vi "Server_Globals.vi"() -> ()   [LabVIEW 2011]
doc: "The Server_Globals vi contain global variables used within the server software."
panel:
  out "External Settings":T1
  in  "Session Settings":T2={"I/O Settings"=[0, 0, 0, 0, 0, 0, 0, 0, 0, 0, 0, 0, 0, 0, 0, 0, 0], "Instrument Handle"={"5402"="", " 5112"="", "4072"="", "USB"="", "4110"=""}, "Logfile"=refnum, "Log Level"=0, "Clear"=[], "OS Set"={"instrument handle out"="", "remaining string"="", "Settings"={"Horizontal Conf."={"Min. Sample rate"=0.0, "Reference position"=0.0, "Record Length"=0}, "Channel A"={"Enable"=FALSE, "Vertical coupling"=0.0, "Vertical range"=0.0, "Vertical offset"=0.0, "Probe attenuation"=1.0}, "Channel B"={"Enable"=FALSE, "Vertical coupling"=0.0, "Vertical range"=0.0, "Vertical offset"=0.0, "Probe attenuation"=1.0}, "Trigger"={"Source"=enum."channel 1", "Slope"=enum."Positive", "Coupling"=enum."AC", "Level"=0.0, "Holdoff"=0.0, "Delay"=0.0, " Timeout"=0.0, " Mode"=enum."Normal"}, "Measurements"={"Measurement 1, Channel"=enum."Channel 1", "Measurement 1, Selection"=0, "Measurement 2, Channel"=enum."Channel 1", "Measurement 2,  Selection"=0, "Measurement 3, Channel"=enum."Channel 1", "Measurement 3, Selection 3"=0}}}, "DC Power Supply"={"0"="", "1"="", "2"="", "3"="", "4"=""}, "USB Interface"={"0"="", "1"="", "2"="", "3"="", "4"=""}, "Function Generator"={"0"="", "1"="", "2"="", "3"="", "4"=""}, "Digital Multimeter"={"0"="", "1"="", "2"="", "3"="", "4"=""}, "Digital Osciliscope"={"0"="", "1"="", "2"="", "3"="", "4"=""}, "To M Server"="", "Adres"=[], "Matrix version"="", "MD5"="", "Digital Multimeter Card 2"={"0"="", "1"="", "2"="", "3"="", "4"=""}} {"I/O Settings" format="%032b"}
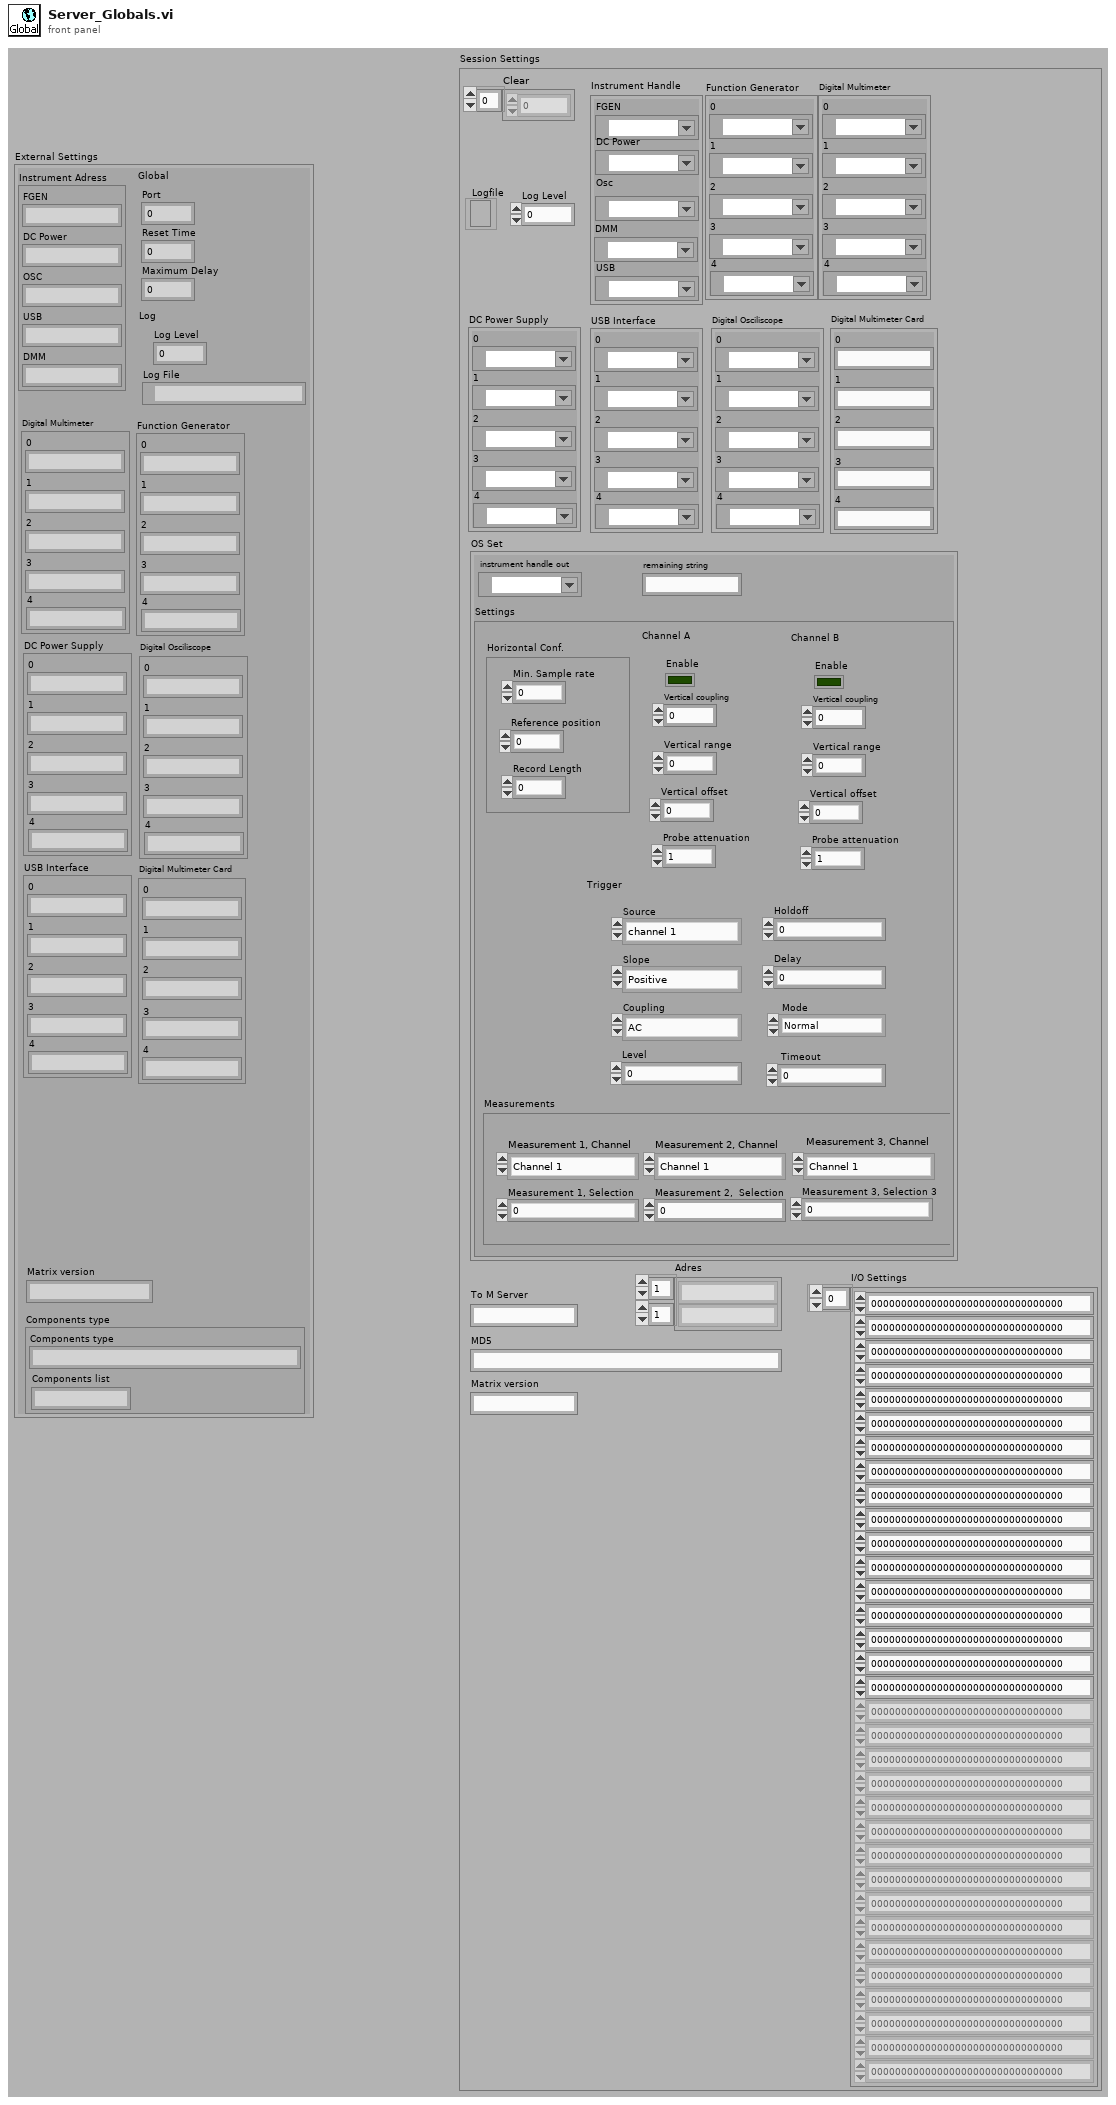
[diagram p1: front panel]
types:
  T1 = cluster{"Global":cluster{"Port":i32, "Reset Time":i32, "Maximum Delay":i32}, "Instrument Adress":cluster{"FGEN":string, "DC Power":string, "OSC":string, "USB":string, "DMM":string}, "Log":cluster{"Log Level":u32, "Log File":path}, "Digital Multimeter":cluster{"0":string, "1":string, "2":string, "3":string, "4":string}, "Function Generator":cluster{"0":string, "1":string, "2":string, "3":string, "4":string}, "Digital Osciliscope":cluster{"0":string, "1":string, "2":string, "3":string, "4":string}, "DC Power Supply":cluster{"0":string, "1":string, "2":string, "3":string, "4":string}, "USB Interface":cluster{"0":string, "1":string, "2":string, "3":string, "4":string}, "Components type":cluster{"Components type":string, "Components list":string}, "Matrix version":string, "Digital Multimeter Card 2":cluster{"0":string, "1":string, "2":string, "3":string, "4":string}}
  T2 = cluster{"I/O Settings":u64[], "Instrument Handle":cluster{"5402":refnum<k15>, " 5112":refnum<k15>, "4072":refnum<k15>, "USB":refnum<visa-resource-name>, "4110":refnum<k15>}, "Logfile":refnum<file>, "Log Level":i8, "Clear":i32[], "OS Set":cluster{"instrument handle out":refnum<k15>, "remaining string":string, "Settings":cluster{"Horizontal Conf.":cluster{"Min. Sample rate":dbl, "Reference position":dbl, "Record Length":i16}, "Channel A":cluster{"Enable":bool, "Vertical coupling":dbl, "Vertical range":dbl, "Vertical offset":dbl, "Probe attenuation":dbl}, "Channel B":cluster{"Enable":bool, "Vertical coupling":dbl, "Vertical range":dbl, "Vertical offset":dbl, "Probe attenuation":dbl}, "Trigger":cluster{"Source":enum8{"channel 1", "channel 2", "Imediate", "External trigger"}, "Slope":enum8{"Positive", "Negative"}, "Coupling":enum8{"AC", "DC"}, "Level":dbl, "Holdoff":dbl, "Delay":dbl, " Timeout":dbl, " Mode":enum8{"Normal", "Auto", "Auto Level"}}, "Measurements":cluster{"Measurement 1, Channel":enum8{"Channel 1", "Channel 2", "Channel 3", "Channel 4"}, "Measurement 1, Selection":u16, "Measurement 2, Channel":enum8{"Channel 1", "Channel 2", "Channel 3", "Channel 4"}, "Measurement 2,  Selection":u16, "Measurement 3, Channel":enum8{"Channel 1", "Channel 2", "Channel 3", "Channel 4"}, "Measurement 3, Selection 3":u16}}}, "DC Power Supply":cluster{"0":refnum<k15>, "1":refnum<k15>, "2":refnum<k15>, "3":refnum<k15>, "4":refnum<k15>}, "USB Interface":cluster{"0":refnum<visa-resource-name>, "1":refnum<visa-resource-name>, "2":refnum<visa-resource-name>, "3":refnum<visa-resource-name>, "4":refnum<visa-resource-name>}, "Function Generator":cluster{"0":refnum<k15>, "1":refnum<k15>, "2":refnum<k15>, "3":refnum<k15>, "4":refnum<k15>}, "Digital Multimeter":cluster{"0":refnum<k15>, "1":refnum<k15>, "2":refnum<k15>, "3":refnum<k15>, "4":refnum<k15>}, "Digital Osciliscope":cluster{"0":refnum<k15>, "1":refnum<k15>, "2":refnum<k15>, "3":refnum<k15>, "4":refnum<k15>}, "To M Server":string, "Adres":string[][], "Matrix version":string, "MD5":string, "Digital Multimeter Card 2":cluster{"0":string, "1":string, "2":string, "3":string, "4":string}}
diagram:
